vi "AerotechGUI.vi"() -> ()   [LabVIEW 2009, in "Aerotech.lvlib"]
uses:
  Aerotech.lvlib
  Controls/AerotechTarget.ctl
panel:
  out "AEROTECH.TARGET":T1
  in  "Position":dbl
  in  "POSITION Button":bool
  in  "HOME button":bool
  in  "QUIT Button":bool
  in  "IDLE Button":bool
  in  "TRACK Button":bool
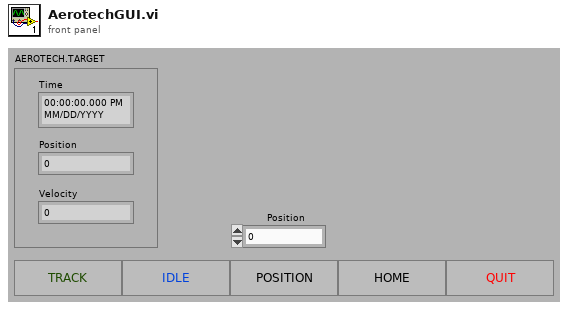
[diagram p1: front panel]
types:
  T1 = typedef "AerotechTarget.ctl" = cluster{"Time":timestamp, "Position":dbl, "Velocity":dbl}
  T2 = typedef "AerotechState.ctl" = enum16{"INITING", "IDLING", "SLEWING", "TRACKING", "MOVING", "HOMING", "STOPPING"}
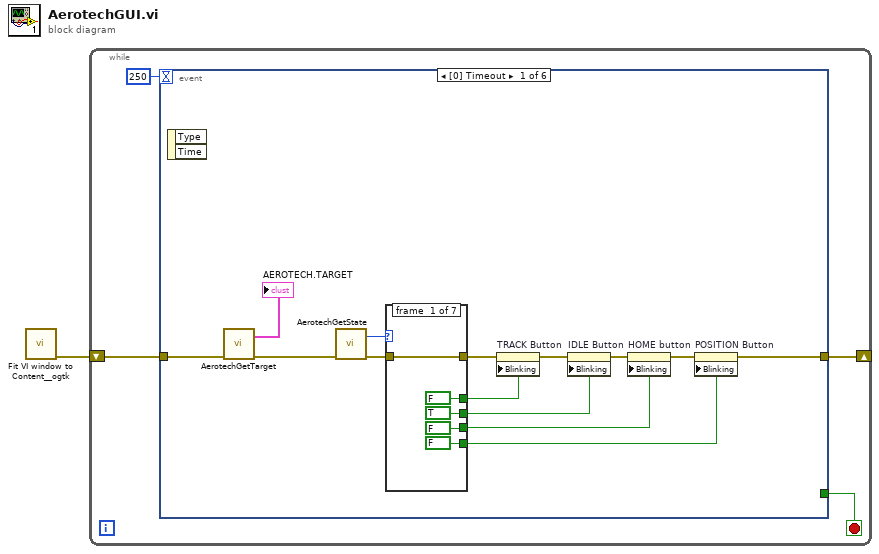
[diagram p0: block diagram]
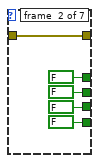
[diagram p2: hidden frame]
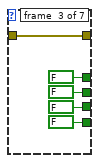
[diagram p3: hidden frame]
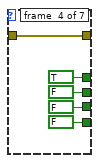
[diagram p4: hidden frame]
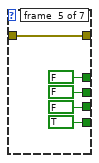
[diagram p5: hidden frame]
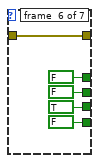
[diagram p6: hidden frame]
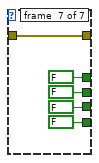
[diagram p7: hidden frame]
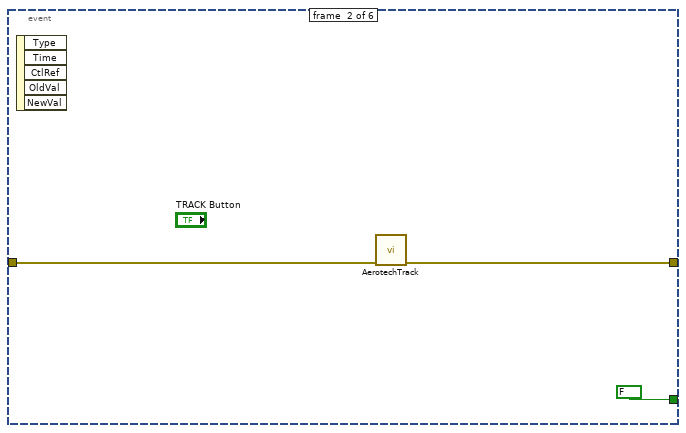
[diagram p8: hidden frame]
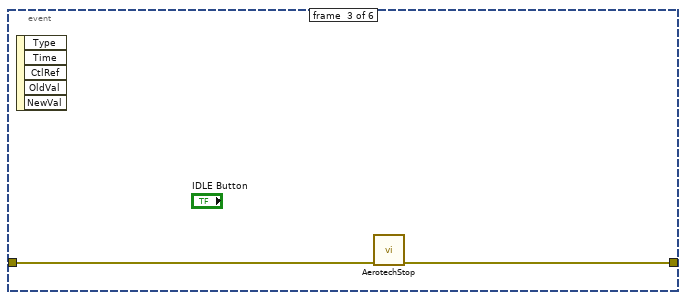
[diagram p9: hidden frame]
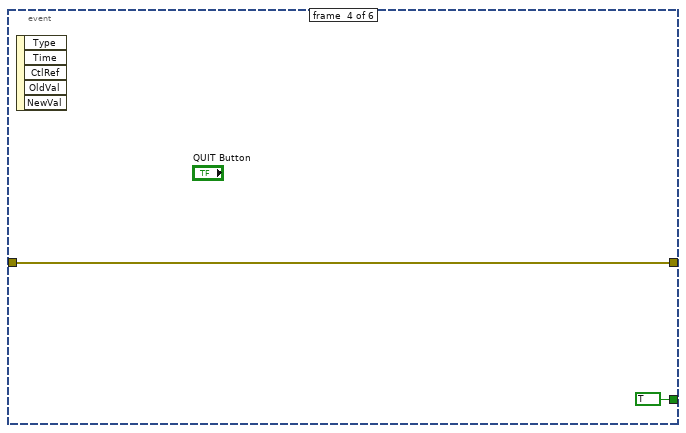
[diagram p10: hidden frame]
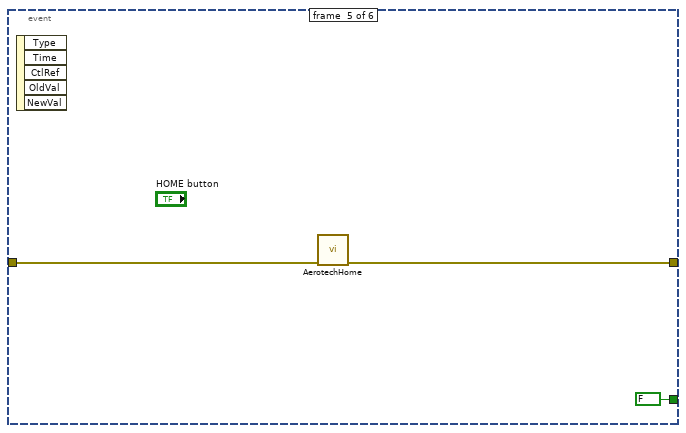
[diagram p11: hidden frame]
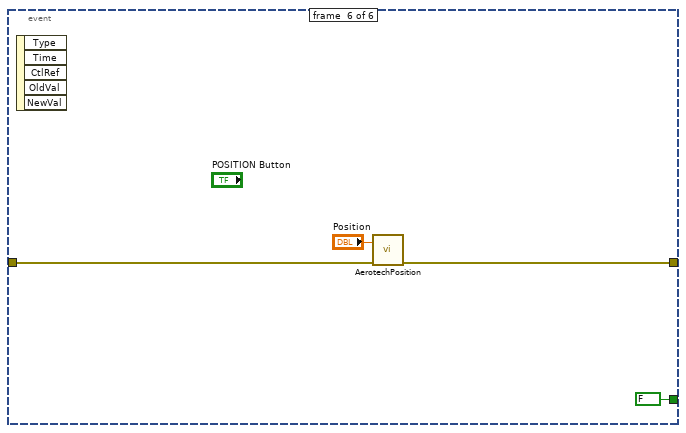
[diagram p12: hidden frame]
diagram:
  n1 = call <userlib>:"Fit VI window to Content__ogtk.vi"() -> ("error out"=w1:errorcluster)  [unwired: 6 in, 1 out]
  n2 = while {
    shift-right: [w4] -> _
    shift-left: w1 -> [w5]
    stop <- w2 stop-if-true
    n3 = event shown="[0] Timeout" {
      selector: _ -> [_ _ _ _ _ _]
      dyn-events: _ -> [_ _ _ _ _ _]
      timeout: 250 -> [_ _ _ _ _ _]
      tunnel: w5 -> [w8 w57 w59 w61 w64 w68]
      tunnel: [w16 w56 w58 w61 w63 w67] -> w4
      tunnel: [_ FALSE _ TRUE FALSE FALSE] -> w2
      event #0 {
        n4 = event-data() -> ()  [unwired: 1 in, 2 out]
        n5 = call "AerotechGetTarget.vi"("error in (no error)"=w8) -> ("error out"=w7:errorcluster, "AEROTECH.TARGET"=→"AEROTECH.TARGET":T1)  [unwired: 3 in]
        n6 = call "AerotechGetState.vi"("error in (no error)"=w7) -> ("error out"=w15:errorcluster, "State"=w14:T2)  [unwired: 3 in]
        n7 = case shown="\"HOMING\"" w14 {
          tunnel: w15 -> [w24 w29 w34 w39 w44 w49 w54]
          tunnel: [w24 w29 w34 w39 w44 w49 w54] -> w13
          tunnel: [FALSE FALSE FALSE TRUE FALSE FALSE FALSE] -> w12
          tunnel: [TRUE FALSE FALSE FALSE FALSE FALSE FALSE] -> w11
          tunnel: [FALSE FALSE FALSE FALSE FALSE TRUE FALSE] -> w10
          tunnel: [FALSE FALSE FALSE FALSE TRUE FALSE FALSE] -> w9
          frame #0 {
          }
          frame #1 {
          }
          frame #2 {
          }
          frame #3 {
          }
          frame #4 {
          }
          frame #5 {
          }
          frame #6 {
          }
        }
        n8 = property on="TRACK Button" class="Bool"(error in=w13, "Blinking"=w12) -> (error out=w19:errorcluster)  [unwired: 1 in, 1 out]
        n9 = property on="IDLE Button" class="Bool"(error in=w19, "Blinking"=w11) -> (error out=w18:errorcluster)  [unwired: 1 in, 1 out]
        n10 = property on="HOME button" class="Bool"(error in=w18, "Blinking"=w10) -> (error out=w17:errorcluster)  [unwired: 1 in, 1 out]
        n11 = property on="POSITION Button" class="Bool"(error in=w17, "Blinking"=w9) -> (error out=w16:errorcluster)  [unwired: 1 in, 1 out]
      }
      event #1 {
        n12 = event-data() -> ()  [unwired: 1 in, 5 out]
        n13 = call "AerotechTrack.vi"("error in (no error)"=w57) -> ("error out"=w56:errorcluster)  [unwired: 10 in]
      }
      event #2 {
        n14 = event-data() -> ()  [unwired: 1 in, 5 out]
        n15 = call "AerotechStop.vi"("error in (no error)"=w59) -> ("error out"=w58:errorcluster)  [unwired: 10 in]
      }
      event #3 {
        n16 = event-data() -> ()  [unwired: 1 in, 5 out]
      }
      event #4 {
        n17 = event-data() -> ()  [unwired: 1 in, 5 out]
        n18 = call "AerotechHome.vi"("error in (no error)"=w64) -> ("error out"=w63:errorcluster)  [unwired: 10 in]
      }
      event #5 {
        n19 = event-data() -> ()  [unwired: 1 in, 5 out]
        n20 = call "AerotechPosition.vi"("error in (no error)"=w68, "Position"="Position") -> ("error out"=w67:errorcluster)  [unwired: 3 in]
      }
    }
  }
